vi "stimulate_and_record_async.vi"(3 "SSH password":string, 4 "Transfer and Run Date Folder After Experiment":bool, 5 "SSH user name":string, 6 "Tags":string, 7 "Frames":i32, 8 "Convert Power to Voltage":bool, 9 "voltages/power":dbl[](array[numeric]), 10 "parameters":string[](array[string]), 11 "parameters headers":string[](array[string])) -> ()   [LabVIEW 2014]
uses:
  <vilib>/vision/driver/IMAQdx.llb/IMAQdx Acquisition Mode.ctl
  <vilib>/userdefined/High Color/IMAQdx.ctl
  <vilib>/vision/driver/IMAQdx.llb/IMAQdx Buffer Number Mode.ctl
  <vilib>/Utility/file.llb/Write To Spreadsheet File (DBL).vi
  <vilib>/Utility/file.llb/Write To Spreadsheet File (string).vi
  <vilib>/Utility/file.llb/Read From Spreadsheet File (string).vi
  <vilib>/vision/driver/NI_Vision_Acquisition_Software.lvlib
panel:
  out "Saved Buffer Number":u32
  out "ProcessFrameRate":dbl
  out "# elements in queue":i32
  out "CameraFrameRate":dbl
  out "Camera Buffer Number":u32
  out "Image":T1(plugin-control)
  out "JPEG Quality":dbl
  out "Error":string
  out "Save Directory":path
  in  "stop":bool
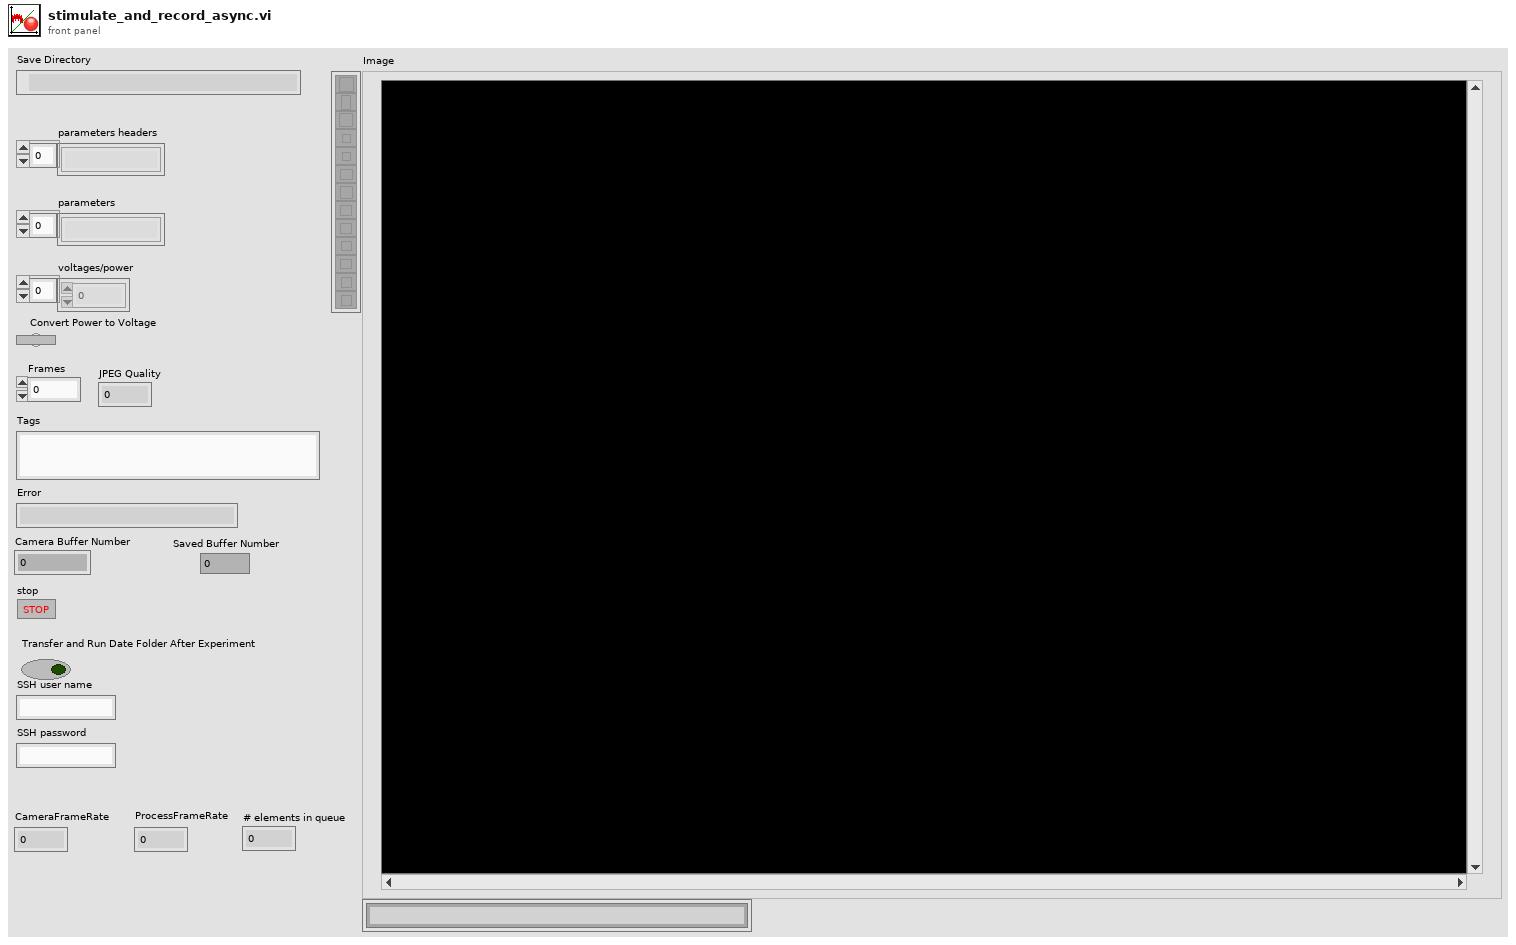
[diagram p1: front panel]
types:
  T1 = typedef "IMAQ Image.ctl" = refnum<image>
  T2 = typedef "IMAQdx.ctl" = refnum<k21>
  T3 = typedef "NI_Vision_Acquisition_Software.lvlib/IMAQdx Buffer Number Mode.ctl" = enum32{"Next", "Last", "Buffer Number"}
  T4 = typedef "Image Type" = u32
  T5 = typedef "NI_Vision_Acquisition_Software.lvlib/IMAQdx Acquisition Mode.ctl" = enum32{"One Shot", "Continuous"}
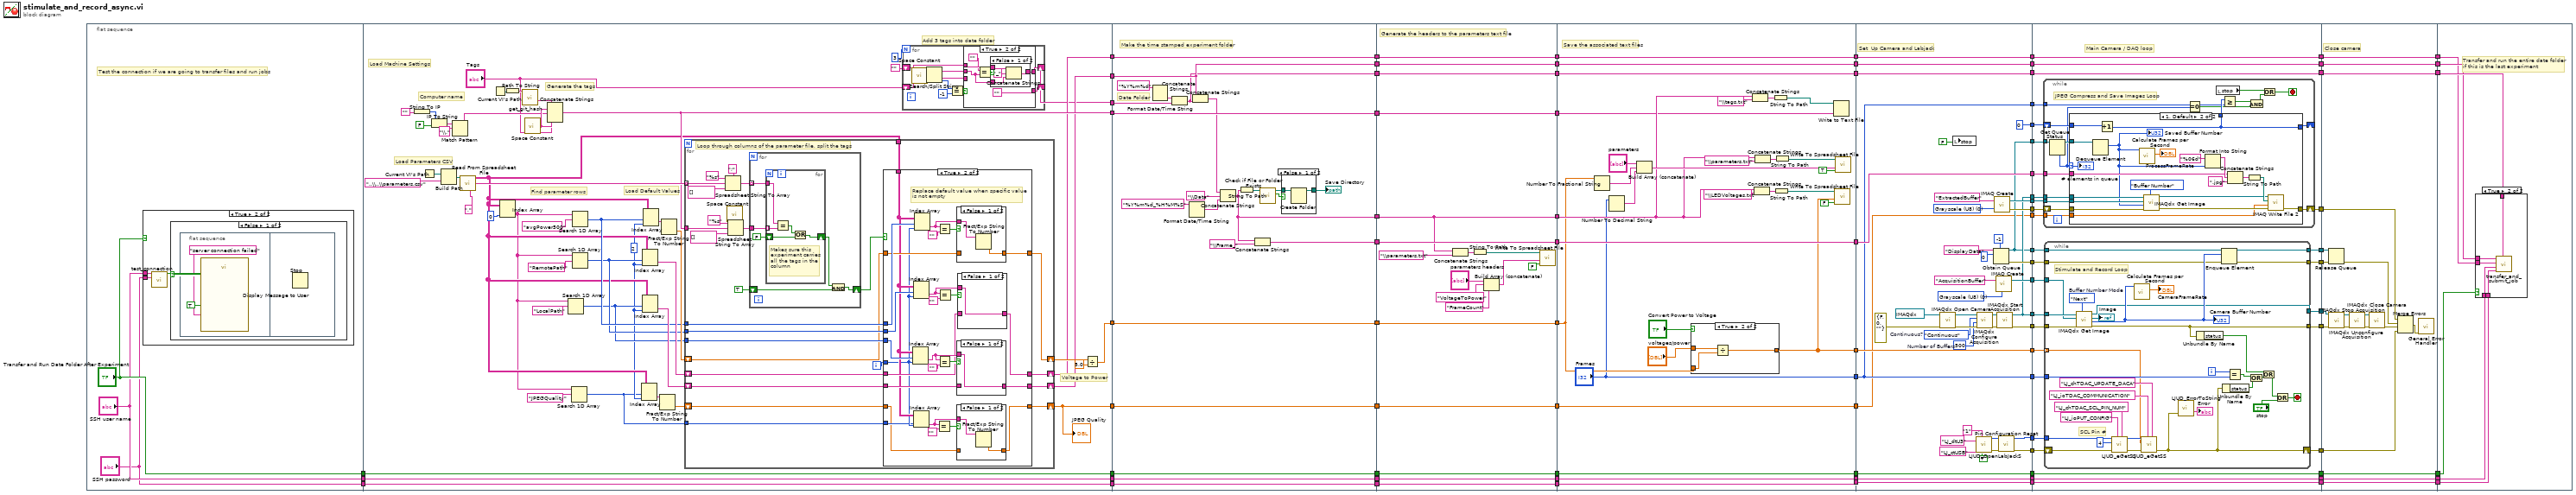
[diagram p0: block diagram]
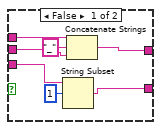
[diagram p4: hidden frame]
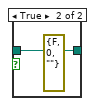
[diagram p11: hidden frame]
diagram:
  n1 = flat-sequence {
    tunnel: ["Transfer and Run Date Folder After Experiment"] -> w48
    tunnel: ["SSH user name"] -> w47
    tunnel: ["SSH password"] -> w46
    tunnel: [w132] -> w78
    tunnel: [w115] -> w77
    tunnel: [w106] -> w68
    tunnel: [w107] -> w67
    tunnel: w48 -> [w124]
    tunnel: w47 -> [w123]
    tunnel: w46 -> [w122]
    tunnel: [w124] -> w39
    tunnel: [w123] -> w32
    tunnel: [w122] -> w31
    tunnel: [w103] -> w24
    tunnel: [w94] -> w23
    tunnel: [w268] -> w62
    tunnel: [w267] -> w60
    tunnel: [w266] -> w58
    tunnel: [w265] -> w56
    tunnel: [w247] -> w54
    tunnel: [w249] -> w52
    tunnel: [w264] -> w50
    tunnel: w67 -> [w264]
    tunnel: w68 -> [w249]
    tunnel: w77 -> [w265]
    tunnel: w78 -> [w266]
    tunnel: [w256] -> w40
    tunnel: w39 -> [w256]
    tunnel: [w255] -> w33
    tunnel: w32 -> [w255]
    tunnel: w31 -> [w254]
    tunnel: [w254] -> w30
    tunnel: w24 -> [w250]
    tunnel: w23 -> [w246]
    tunnel: [w246] -> w20
    tunnel: w62 -> [w290]
    tunnel: [w290] -> w61
    tunnel: w60 -> [w276]
    tunnel: [w276] -> w59
    tunnel: w58 -> [w289]
    tunnel: [w289] -> w57
    tunnel: w56 -> [w288]
    tunnel: [w288] -> w55
    tunnel: w54 -> [w287]
    tunnel: [w287] -> w53
    tunnel: w52 -> [w286]
    tunnel: [w286] -> w51
    tunnel: w50 -> [w285]
    tunnel: [w285] -> w49
    tunnel: [w275] -> w41
    tunnel: w40 -> [w275]
    tunnel: [w274] -> w34
    tunnel: w33 -> [w274]
    tunnel: w30 -> [w273]
    tunnel: [w273] -> w29
    tunnel: [w272] -> w21
    tunnel: w20 -> [w272]
    tunnel: w61 -> [w318]
    tunnel: [w318] -> w83
    tunnel: [w301] -> w81
    tunnel: ["Frames"] -> w80
    tunnel: w59 -> [w310]
    tunnel: w57 -> [w297]
    tunnel: w55 -> [w292]
    tunnel: w53 -> [w306]
    tunnel: [w306] -> w73
    tunnel: [w305] -> w69
    tunnel: w51 -> [w305]
    tunnel: [w304] -> w63
    tunnel: w49 -> [w304]
    tunnel: [w295] -> w42
    tunnel: w41 -> [w295]
    tunnel: [w294] -> w35
    tunnel: w34 -> [w294]
    tunnel: w29 -> [w293]
    tunnel: [w293] -> w28
    tunnel: [w291] -> w22
    tunnel: w21 -> [w291]
    tunnel: w83 -> [w330]
    tunnel: [w360] -> w85
    tunnel: [w359] -> w84
    tunnel: [w363] -> w82
    tunnel: w81 -> [w363]
    tunnel: w80 -> [w329]
    tunnel: [w329] -> w79
    tunnel: [w357] -> w74
    tunnel: w73 -> [w357]
    tunnel: [w356] -> w70
    tunnel: w69 -> [w356]
    tunnel: [w355] -> w64
    tunnel: w63 -> [w355]
    tunnel: [w354] -> w43
    tunnel: w42 -> [w354]
    tunnel: [w353] -> w36
    tunnel: w35 -> [w353]
    tunnel: w28 -> [w352]
    tunnel: [w352] -> w27
    tunnel: w22 -> [w327]
    tunnel: [w336] -> w19
    tunnel: [w331] -> w18
    tunnel: [w335] -> w17
    tunnel: [w334] -> w16
    tunnel: [w328] -> w15
    tunnel: [w333] -> w12
    tunnel: [w332] -> w11
    tunnel: [w331] -> w10
    tunnel: [w330] -> w9
    tunnel: [w329] -> w8
    tunnel: [w328] -> w7
    tunnel: [w327] -> w6
    tunnel: [0] -> w2
    tunnel: w85 -> [w395]
    tunnel: w84 -> [w394]
    tunnel: w82 -> [w393]
    tunnel: w79 -> [w392]
    tunnel: [w391] -> w75
    tunnel: w74 -> [w391]
    tunnel: [w390] -> w71
    tunnel: w70 -> [w390]
    tunnel: [w389] -> w65
    tunnel: w64 -> [w389]
    tunnel: [w388] -> w44
    tunnel: w43 -> [w388]
    tunnel: [w387] -> w37
    tunnel: w36 -> [w387]
    tunnel: w27 -> [w386]
    tunnel: [w386] -> w26
    tunnel: w19 -> [w385]
    tunnel: w18 -> [w384]
    tunnel: w17 -> [w383]
    tunnel: w16 -> [w382]
    tunnel: w15 -> [w381]
    tunnel: [w380] -> w14
    tunnel: [w379] -> w13
    tunnel: w12 -> [w378]
    tunnel: w11 -> [w377]
    tunnel: w10 -> [w376]
    tunnel: w9 -> [w375]
    tunnel: w8 -> [w374]
    tunnel: w7 -> [w373]
    tunnel: w6 -> [w372]
    tunnel: [w371] -> w5
    tunnel: [w368] -> w4
    tunnel: [w370] -> w3
    tunnel: w2 -> [w369]
    tunnel: [w367] -> w1
    tunnel: [w487] -> w76
    tunnel: w75 -> [w487]
    tunnel: [w486] -> w72
    tunnel: w71 -> [w486]
    tunnel: [w485] -> w66
    tunnel: w65 -> [w485]
    tunnel: [w484] -> w45
    tunnel: w44 -> [w484]
    tunnel: [w483] -> w38
    tunnel: w37 -> [w483]
    tunnel: w26 -> [w482]
    tunnel: [w482] -> w25
    tunnel: w14 -> [w477]
    tunnel: w13 -> [w476]
    tunnel: w5 -> [w473]
    tunnel: w4 -> [w472]
    tunnel: w3 -> [w471]
    tunnel: w1 -> [w470]
    tunnel: w76 -> [w493]
    tunnel: w72 -> [w492]
    tunnel: w66 -> [w491]
    tunnel: w45 -> [w490]
    tunnel: w38 -> [w489]
    tunnel: w25 -> [w488]
    frame #0 {
      # "Test the connection if we are going to transfer files and run jobs"
      n2 = case shown="True" "Transfer and Run Date Folder After Experiment" {
        tunnel: "SSH password" -> [_ w91]
        tunnel: "SSH user name" -> [_ w89]
        frame False {
        }
        frame True {
          n3 = call "test_connection.vi"("Username"=w89, "Password"=w91) -> ("Connection Successful"=w90:bool)  [unwired: 7 in]
          n4 = case shown="False" w90 {
            frame False {
              n5 = flat-sequence {
                frame #0 {
                  n6 = call "Display Message to User"("Enable"=TRUE, "Message"="server connection failed") -> ()  [unwired: 8 in, 2 out]
                }
                frame #1 {
                  n7 = Stop() -> ()  [unwired: 1 in]
                }
              }
            }
            frame True {
            }
          }
        }
      }
    }
    frame #1 {
      w97 = 2
      # "Add 3 tags into date folder"
      # "Generate the tags"
      # "Find parameter rows"
      # "Load Default Values"
      # "Voltage to Power"
      # "Load Parameters CSV"
      # "Computer name"
      # "Load Machine Settings"
      n8 = String To IP(1:"") -> (0:w140:u32)
      n9 = Current VI's Path() -> (path=w135:path)
      n10 = IP To String(1:FALSE, 2:w140) -> (0:w137:string)
      n11 = Build Path(base path=w135, name or relative path="..\\..\\parameters.csv") -> (appended path=w126:path)
      n12 = Match Pattern(string=w137, regular expression="\\.") -> (before substring=w117:string)  [unwired: 1 in, 3 out]
      n13 = call-poly <vilib>:"Read From Spreadsheet File.vi"("delimiter (\\t)"=",", "file path (dialog if empty)"=w126) -> ("first row"=w116:string[], "all rows"=w99:string[][])  [unwired: 5 in, 3 out]
      n14 = Current VI's Path() -> (path=w119:path)
      n15 = Index Array(array=w99, index (col)=0) -> (element=w98:string[])  [unwired: 1 in]
      n16 = Path To String(path=w119) -> (string=w118:string)
      n17 = call "get_git_hash.vi"("VI folder"=w118) -> ("github hash"=w121:string)  [unwired: 10 in]
      n18 = call <vilib>:"Space Constant.vi"() -> ("String"=w120:string)
      n19 = Concatenate Strings(w121, w120, w117, w120, "Tags") -> (w115:string)
      n20 = Search 1D Array(1D array=w98, element="LocalPath") -> (index of element=w109:i32)  [unwired: 1 in]
      n21 = Search 1D Array(1D array=w98, element="JPEGQuality") -> (index of element=w95:i32)  [unwired: 1 in]
      n22 = Search 1D Array(1D array=w98, element="RemotePath") -> (index of element=w110:i32)  [unwired: 1 in]
      n23 = Search 1D Array(1D array=w98, element="avgPower500") -> (index of element=w111:i32)  [unwired: 1 in]
      n24 = Index Array(array=w99, index (row)=w95, index (col)=w97) -> (element=w100:string)
      n25 = Index Array(array=w99, index (row)=w110, index (col)=w97) -> (element=w113:string)
      n26 = Index Array(array=w99, index (row)=w109, index (col)=w97) -> (element=w112:string)
      n27 = Index Array(array=w99, index (row)=w111, index (col)=w97) -> (element=w128:string)
      n28 = Fract/Exp String To Number(string=w100) -> (number=w96:dbl)  [unwired: 3 in, 1 out]
      n29 = Fract/Exp String To Number(string=w128) -> (number=w114:dbl)  [unwired: 3 in, 1 out]
      n30 = for {
        tunnel: w116 -> [w194] mode=indexing
        tunnel: w115 -> [w186]
        tunnel: w111 -> [w181]
        tunnel: w110 -> [w180]
        tunnel: w109 -> [w179]
        tunnel: w99 -> [w184]
        shift-right: [w176] -> w108
        shift-left: w114 -> [w177]
        shift-right: [w173] -> w107
        shift-left: w113 -> [w174]
        shift-right: [w172] -> w106
        shift-left: w112 -> [w175]
        shift-right: [w169] -> w94
        shift-left: w96 -> [w171]
        tunnel: w95 -> [w170]
        i -> [w178]
        # "Loop through columns of the parameter file, split the tags"
        n31 = Spreadsheet String To Array(delimiter (Tab)=";", format string="%s", spreadsheet string=w194, array type (2D Dbl)=string[] []) -> (array=w190:string[])
        n32 = call <vilib>:"Space Constant.vi"() -> ("String"=w188:string)
        n33 = Spreadsheet String To Array(delimiter (Tab)=w188, format string="%s", spreadsheet string=w186, array type (2D Dbl)=string[] []) -> (array=w185:string[])
        n34 = for {
          tunnel: w190 -> [w240] mode=indexing
          tunnel: w185 -> [w239]
          shift-right: [w237] -> w182
          shift-left: TRUE -> [w235]
          n35 = for {
            tunnel: w240 -> [w245]
            tunnel: w239 -> [w244] mode=indexing
            shift-right: [w241] -> w236
            shift-left: FALSE -> [w242]
            # "Makes sure this\nexperiment carries\nall the tags in the\ncolumn"
            n36 = Equal?(x=w245, y=w244) -> (x = y?=w243:bool)
            n37 = Or(x=w243, y=w242) -> (x .or. y?=w241:bool)
          }
          n38 = And(x=w236, y=w235) -> (x .and. y?=w237:bool)
        }
        n39 = case shown="True" w182 {
          tunnel: w177 -> [w198 w219]
          tunnel: [w198 w218] -> w176
          tunnel: w181 -> [_ w224]
          tunnel: w180 -> [_ w223]
          tunnel: w179 -> [_ w222]
          tunnel: w178 -> [_ w201]
          tunnel: w184 -> [_ w202]
          tunnel: [w197 w208] -> w173
          tunnel: [w196 w210] -> w172
          tunnel: w175 -> [w196 w209]
          tunnel: w174 -> [w197 w207]
          tunnel: w171 -> [w195 w199]
          tunnel: w170 -> [_ w200]
          tunnel: [w195 w203] -> w169
          frame False {
          }
          frame True {
            # "Replace default value when specific value\nis not empty"
            n40 = Index Array(array=w202, index (row)=w222, index (col)=w201) -> (element=w211:string)
            n41 = Index Array(array=w202, index (row)=w223, index (col)=w201) -> (element=w214:string)
            n42 = Index Array(array=w202, index (row)=w200, index (col)=w201) -> (element=w204:string)
            n43 = Index Array(array=w202, index (row)=w224, index (col)=w201) -> (element=w217:string)
            n44 = Equal?(x=w204, y="") -> (x = y?=w205:bool)
            n45 = Equal?(x=w217, y="") -> (x = y?=w220:bool)
            n46 = Equal?(x=w211, y="") -> (x = y?=w212:bool)
            n47 = Equal?(x=w214, y="") -> (x = y?=w215:bool)
            n48 = case shown="False" w205 {
              tunnel: w199 -> [_ w227]
              tunnel: [w226 w227] -> w203
              tunnel: w204 -> [w225 _]
              frame False {
                n49 = Fract/Exp String To Number(string=w225) -> (number=w226:dbl)  [unwired: 3 in, 1 out]
              }
              frame True {
              }
            }
            n50 = case shown="False" w220 {
              tunnel: w219 -> [_ w234]
              tunnel: [w233 w234] -> w218
              tunnel: w217 -> [w232 _]
              frame False {
                n51 = Fract/Exp String To Number(string=w232) -> (number=w233:dbl)  [unwired: 3 in, 1 out]
              }
              frame True {
              }
            }
            n52 = case shown="False" w212 {
              tunnel: w211 -> [w228 _]
              tunnel: [w228 w229] -> w210
              tunnel: w209 -> [_ w229]
              frame False {
              }
              frame True {
              }
            }
            n53 = case shown="False" w215 {
              tunnel: w214 -> [w230 _]
              tunnel: [w230 w231] -> w208
              tunnel: w207 -> [_ w231]
              frame False {
              }
              frame True {
              }
            }
          }
        }
      }
      "JPEG Quality" <- w94
      n54 = for {
        N: 3 -> [_]
        shift-right: [w141] -> _
        shift-left: "Tags" -> [w150]
        shift-right: [w143] -> w103
        shift-left: "" -> [w148]
        n55 = call <vilib>:"Space Constant.vi"() -> ("String"=w149:string)
        n56 = Search/Split String(string=w150, search string/char (-)=w149) -> (substring before match=w147:string, match + rest of string=w146:string, offset of match=w145:i32)  [unwired: 1 in]
        n57 = Equal?(x=w145, y=-1) -> (x = y?=w142:bool)
        n58 = case shown="True" w142 {
          tunnel: w148 -> [w151 w161]
          tunnel: w147 -> [w152 w158]
          tunnel: w146 -> [w153 _]
          tunnel: [w155 ""] -> w141
          tunnel: [w154 w160] -> w143
          frame False {
            n59 = String Subset(string=w153, offset (0)=1) -> (substring=w155:string)  [unwired: 1 in]
            n60 = Concatenate Strings(w151, "_", w152) -> (w154:string)
          }
          frame True {
            n61 = Equal?(x="", y=w158) -> (x = y?=w162:bool)
            n62 = case shown="False" w162 {
              tunnel: w161 -> [w165 w168]
              tunnel: [w166 w168] -> w160
              tunnel: w158 -> [w164 _]
              frame False {
                n63 = Concatenate Strings(w165, "_", w164) -> (w166:string)
              }
              frame True {
              }
            }
          }
        }
      }
      n64 = Divide(x=w108, y=5.0) -> (x/y=w132:dbl)
    }
    frame #2 {
      # "Make the time stamped experiment folder"
      # "Date Folder"
      n65 = Format Date/Time String(time format string (%c)="%Y%m%d") -> (date/time string=w251:string)  [unwired: 2 in]
      n66 = Concatenate Strings(w251, w250) -> (w247:string)
      n67 = Format Date/Time String(time format string (%c)="%Y%m%d_%H%M%S") -> (date/time string=w253:string)  [unwired: 2 in]
      n68 = Concatenate Strings(w249, w247) -> (w248:string)
      n69 = Concatenate Strings(w248, "\\Data", w253) -> (w267:string)
      n70 = String To Path(string=w267) -> (path=w259:path)
      n71 = Concatenate Strings(w267, "\\Frame_") -> (w268:string)
      n72 = call <vilib>:"Check if File or Folder Exists.vi"("path"=w259) -> ("file or folder exists?"=w262:bool, "dup path"=w261:path)  [unwired: 8 in, 1 out]
      n73 = case shown="False" w262 {
        tunnel: [w269 w271] -> w258
        tunnel: w261 -> [w270 w271]
        frame False {
          n74 = Create Folder(path (use dialog)=w270) -> (created path=w269:path)  [unwired: 2 in, 2 out]
        }
        frame True {
          (unwired) errorcluster {"status"=FALSE, "code"=0, "source"=""} ("error out")
        }
      }
      "Save Directory" <- w258
    }
    frame #3 {
      # "Generate the headers to the parameters text file"
      n75 = Concatenate Strings(w276, "\\parameters.txt") -> (w284:string)
      n76 = String To Path(string=w284) -> (path=w283:path)
      n77 = Build Array (concatenate)("parameters headers", "VoltageToPower", "FrameCount") -> (w280:string[])
      n78 = call-poly <vilib>:"Write To Spreadsheet File.vi"("append to file? (new file:F)"=FALSE, "1D data"=w280, "file path (dialog if empty)"=w283) -> ()  [unwired: 5 in, 1 out]
    }
    frame #4 {
      # "Save the associated text files"
      n79 = Number To Fractional String(number=w297) -> (F-format string=w298:string)  [unwired: 3 in]
      n80 = Number To Decimal String(number="Frames") -> (decimal integer string=w299:string)  [unwired: 1 in]
      n81 = Build Array (concatenate)("parameters", w298, w299) -> (w311:string[])
      n82 = case shown="True" "Convert Power to Voltage" {
        tunnel: "voltages/power" -> [w321 w324]
        tunnel: [w321 w322] -> w301
        tunnel: w297 -> [_ w323]
        frame False {
        }
        frame True {
          n83 = Divide(x=w324, y=w323) -> (x/y=w322:dbl[])
        }
      }
      n84 = Concatenate Strings(w310, "\\tags.txt") -> (w308:string)
      n85 = Concatenate Strings(w310, "\\LEDVoltages.txt") -> (w320:string)
      n86 = Concatenate Strings(w310, "\\parameters.txt") -> (w315:string)
      n87 = String To Path(string=w308) -> (path=w307:path)
      n88 = String To Path(string=w320) -> (path=w319:path)
      n89 = String To Path(string=w315) -> (path=w314:path)
      n90 = Write to Text File(file (use dialog)=w307, text=w292) -> ()  [unwired: 2 in, 3 out]
      n91 = call-poly <vilib>:"Write To Spreadsheet File.vi"("append to file? (new file:F)"=FALSE, "1D data"=w301, "file path (dialog if empty)"=w319) -> ()  [unwired: 5 in, 1 out]
      n92 = call-poly <vilib>:"Write To Spreadsheet File.vi"("append to file? (new file:F)"=TRUE, "1D data"=w311, "file path (dialog if empty)"=w314) -> ()  [unwired: 5 in, 1 out]
    }
    frame #5 {
      w339 = T4 0 items=["Grayscale (U8)", "Grayscale (I16)", "Grayscale (SGL)", "Complex (CSG)", "RGB (U32)", "HSL (U32)", "RGB (U64)"] ("Image Type")
      w348 = T4 0 items=["Grayscale (U8)", "Grayscale (I16)", "Grayscale (SGL)", "Complex (CSG)", "RGB (U32)", "HSL (U32)", "RGB (U64)"] ("Image Type")
      w349 = u32 500  # Number of Buffers
      w345 = IMAQdx_Acquisition_Mode."Continuous"  # Continuous?
      # "Set  Up Camera and Labjack"
      n93 = call <vilib>:"IMAQdx Open Camera.vi"("error in"=errorcluster {"status"=FALSE, "code"=0, "source"=""}, "Session In"=T2 "cam0") -> ("error out"=w350:errorcluster, "Session Out"=w351:T2)  [unwired: 8 in]
      n94 = local write "stop"(FALSE) -> ()
      n95 = call "LJUD_OpenLabJackS.vi"("FirstFound"=TRUE, "Address"="1" ("DeviceType"), "ConnectionType"="LJ_ctUSB", "DeviceType"="LJ_dtU3") -> ("error out"=w358:errorcluster, "Handle"=w361:i32)  [unwired: 5 in, 1 out]
      n96 = call <vilib>:"IMAQdx Configure Acquisition.vi"("error in"=w350, "Number of Buffers"=w349, "Continuous?"=w345, "Session In"=w351) -> ("error out"=w346:errorcluster, "Session Out"=w344:T2)  [unwired: 6 in]
      n97 = Obtain Queue(max queue size (-1, unlimited)=-1, name (unnamed)="DisplayData", element data type=u32 0) -> (queue out=w328:refnum<queue>, error out=w334:errorcluster)  [unwired: 2 in, 1 out]
      n98 = call "IMAQ Create"("Image Name"="ExtractedBuffer", "Image Type"=w339) -> ("New Image"=w332:T1, "error out"=w333:errorcluster)  [unwired: 3 in]
      n99 = call "IMAQ Create"("Image Name"="AcquisitionBuffer", "Image Type"=w348) -> ("New Image"=w335:T1)  [unwired: 3 in, 1 out]
      n100 = call <vilib>:"IMAQdx Start Acquisition.vi"("error in"=w346, "Session In"=w344) -> ("error out"=w336:errorcluster, "Session Out"=w331:T2)  [unwired: 8 in]
      n101 = call "Pin Configuration Reset.vi"("error in"=w358, "Handle In"=w361) -> ("error out"=w359:errorcluster, "Handle Out"=w360:i32)  [unwired: 8 in]
    }
    frame #6 {
      # "Main Camera / DAQ loop"
      n102 = while {
        tunnel: w373 -> [w413]
        tunnel: w377 -> [w411]
        tunnel: w376 -> [w410]
        tunnel: w375 -> [w408]
        shift-right: [w407] -> w370
        shift-left: w378 -> [w409]
        tunnel: w374 -> [w400]
        tunnel: w372 -> [w405]
        shift-right: [w402] -> _
        shift-left: w369 -> [w403]
        stop <- w406 stop-if-true
        # "JPEG Compress and Save Images Loop"
        n103 = Get Queue Status(queue=w413) -> (queue out=w412:refnum<queue>, # elements in queue=w396:i32)  [unwired: 2 in, 6 out]
        n104 = case shown="1, Default" w396 {
          selector: w396 -> [_ w434]
          tunnel: w412 -> [_ w432]
          tunnel: w411 -> [_ w431]
          tunnel: w410 -> [_ w430]
          tunnel: w409 -> [w415 w429]
          tunnel: w408 -> [_ w423]
          tunnel: [w415 w419] -> w407
          tunnel: w405 -> [_ w418]
          tunnel: w403 -> [w414 w417]
          tunnel: [w414 w416] -> w402
          tunnel: [w414 w416] -> w401
          frame 0 {
          }
          frame 1, Default {
            n105 = Dequeue Element(queue=w432) -> (element=w420:u32)  [unwired: 2 in, 3 out]
            "Saved Buffer Number" <- w420
            n106 = Increment(x=w417) -> (x+1=w416:i32)
            n107 = call <vilib>:"Calculate Frames per Second.vi"("Buffer Number"=w420) -> ("Processed Frames/s"=→"ProcessFrameRate":dbl)  [unwired: 8 in, 2 out]
            n108 = call <vilib>:"IMAQdx Get Image.vi"("Buffer Number Mode (Next)"=IMAQdx_Buffer_Number_Mode."Buffer Number", "error in"=w429, "Buffer Number In"=w420, "Image In"=w431, "Session In"=w430) -> ("error out"=w421:errorcluster, "Image Out"=w422:T1)  [unwired: 3 in, 2 out]
            n109 = Format Into String(format string="%06d" ("string"), w420) -> (resulting string=w425:string)  [unwired: 2 in, 1 out]
            n110 = Concatenate Strings(w423, w425, ".jpg" ("string")) -> (w427:string)
            n111 = String To Path(string=w427) -> (path=w426:path)
            n112 = call-poly "IMAQ Write File 2"("error in (no error)"=w421, "Image Quality"=w418, "File Path"=w426, "Image"=w422) -> ("error out"=w419:errorcluster)  [unwired: 6 in, 1 out]
            "# elements in queue" <- w434
          }
        }
        n113 = Equal To 0?(x=w396) -> (x = 0?=w397:bool)
        n114 = local read "stop"() -> (w404:bool)
        n115 = Greater Or Equal?(x=w401, y=w400) -> (x >= y?=w399:bool)
        n116 = And(x=w399, y=w397) -> (x .and. y?=w398:bool)
        n117 = Or(x=w404, y=w398) -> (x .or. y?=w406:bool)
      }
      n118 = while {
        tunnel: w395 -> [w454]
        shift-right: [w455] -> w371
        shift-left: w394 -> [w453]
        tunnel: w393 -> [w452] mode=indexing
        tunnel: w392 -> [w463]
        tunnel: w385 -> [w447]
        tunnel: w384 -> [w446]
        tunnel: w383 -> [w445]
        tunnel: w382 -> [w444]
        tunnel: w381 -> [w443]
        tunnel: [w439] -> w367
        tunnel: [w438] -> w368
        tunnel: [w437] -> w380
        tunnel: [w436] -> w379
        i -> [w464]
        stop <- w469 stop-if-true
        w451 = IMAQdx_Buffer_Number_Mode."Next"  # Buffer Number Mode
        # "Stimulate and Record Loop"
        # "SCL Pin #"
        n119 = call <vilib>:"IMAQdx Get Image.vi"("Buffer Number Mode (Next)"=w451, "error in"=w447, "Image In"=w445, "Session In"=w446) -> ("error out"=w436:errorcluster, "Buffer Number Out"=w448:u32, "Image Out"=→"Image":T1, "Session Out"=w437:T2)  [unwired: 4 in]
        "Camera Buffer Number" <- w448
        n120 = call "LJUD_eGetSS.vi"("Channel"="LJ_chTDAC_SCL_PIN_NUM", "IOType"="LJ_ioPUT_CONFIG", "error in"=w453, "Value Write"=4, "Handle In"=w454) -> ("error out"=w456:errorcluster, "Handle Out"=w459:i32)  [unwired: 4 in, 1 out]
        n121 = call <vilib>:"Calculate Frames per Second.vi"("Buffer Number"=w448) -> ("Processed Frames/s"=→"CameraFrameRate":dbl)  [unwired: 8 in, 2 out]
        n122 = call "LJUD_eGetSS.vi"("Channel"="LJ_chTDAC_UPDATE_DACA", "IOType"="LJ_ioTDAC_COMMUNICATION", "error in"=w456, "Value Write"=w452, "Handle In"=w459) -> ("error out"=w455:errorcluster)  [unwired: 4 in, 2 out]
        n123 = call "LJUD_ErrorToString.vi"("error in"=w455) -> ("String"=→"Error":string)  [unwired: 10 in]
        n124 = Unbundle By Name(w436) -> ("status"=w442:bool)
        n125 = Enqueue Element(queue=w443, element=w448, error in (no error)=w444) -> (queue out=w439:refnum<queue>, error out=w438:errorcluster)  [unwired: 1 in, 1 out]
        n126 = Unbundle By Name(w455) -> ("status"=w466:bool)
        n127 = Equal?(x=w464, y=w463) -> (x = y?=w465:bool)
        n128 = Or(x=w465, y=w466) -> (x .or. y?=w441:bool)
        n129 = Or(x=w442, y=w441) -> (x .or. y?=w440:bool)
        n130 = Or(x=w440, y="stop") -> (x .or. y?=w469:bool)
      }
    }
    frame #7 {
      # "Close camera"
      n131 = Release Queue(queue=w470) -> ()  [unwired: 2 in, 3 out]
      n132 = call <vilib>:"IMAQdx Stop Acquisition.vi"("error in"=w476, "Session In"=w477) -> ("error out"=w478:errorcluster, "Session Out"=w479:T2)  [unwired: 8 in]
      n133 = call <vilib>:"IMAQdx Unconfigure Acquisition.vi"("error in"=w478, "Session In"=w479) -> ("error out"=w481:errorcluster, "Session Out"=w480:T2)  [unwired: 8 in]
      n134 = call <vilib>:"IMAQdx Close Camera.vi"("error in"=w481, "Session In"=w480) -> ("error out"=w474:errorcluster)  [unwired: 9 in]
      n135 = Merge Errors(w471, w472, w474, w473) -> (w475:errorcluster)
      n136 = call <vilib>:"General Error Handler.vi"("error in (no error)"=w475) -> ()  [unwired: 10 in, 5 out]
    }
    frame #8 {
      # "Transfer and run the entire date folder\nif this is the last experiment"
      n137 = case shown="True" w490 {
        tunnel: w493 -> [_ w498]
        tunnel: w492 -> [_ w497]
        tunnel: w491 -> [_ w496]
        tunnel: w489 -> [_ w495]
        tunnel: w488 -> [_ w494]
        frame False {
        }
        frame True {
          n138 = call "transfer_and_submit_job.vi"("Date Folder"=w498, "Password"=w494, "Username"=w495, "Remote Data Directory"=w496, "Local Data Directory"=w497) -> ()  [unwired: 7 in]
        }
      }
    }
  }
